vi "Untitled 2.vi"() -> ()   [LabVIEW 2015]
uses:
  <instrlib>/_niInstr/DSP/v1/Shared/Public/IQ Data.ctl
  <instrlib>/_niInstr/DSP/v1/FPGA/Public/Sub VIs/Fractional Decimator/Fractional Decimator - 1 spc - 2x oc.vi
  <instrlib>/_niInstr/DSP/v1/Xnodes/Public/Decimator/niInstr DSP v1 Decimator FPGA.xnode
  <instrlib>/_niInstr/DSP/v1/Shared/niInstr DSP v1 Shared.lvlib
  <instrlib>/_niInstr/DSP/v1/FPGA/niInstr DSP v1 FPGA.lvlib
panel:
  out "ready for input":bool
  out "output valid":bool
  out "data out":T1
  in  "delay":fxp<+/-,16,0>
  in  "output sample rate":fxp<+,48,1>
  in  "input valid":bool
  in  "reset":bool
  in  "data in":T1
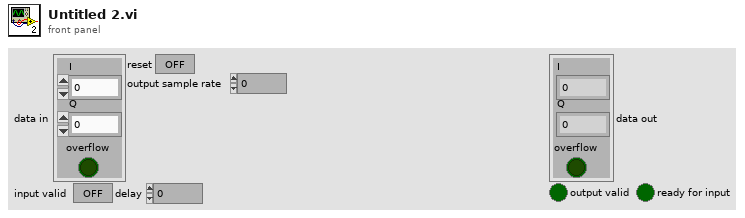
[diagram p1: front panel]
types:
  T1 = typedef "niInstr DSP v1 Shared.lvlib/IQ Data.ctl" = cluster{"I":fxp<+/-,18,1>, "Q":fxp<+/-,18,1>, "overflow":bool}
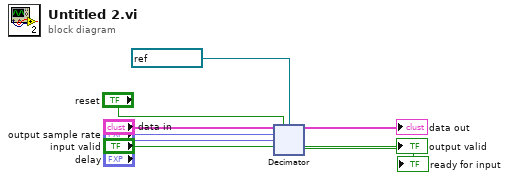
[diagram p0: block diagram]
diagram:
  n1 = xnode "Decimator"("data in"="data in", "reset"="reset", "input valid"="input valid", "output sample rate"="output sample rate", "delay"="delay", "clock x2"=refnum<k21> "204MHz" ("Refnum in")) -> ("data out"=→"data out":T1, "output valid"=→"output valid":bool, "ready for input"=→"ready for input":bool)
